vi "OPC UA SV Server.vi"() -> ()   [LabVIEW 2015]
uses:
  Controls/Folders to Add.ctl
  <vilib>/OPCUA/NI OPC UA Server.lvlib
  Sync Tag Class/Synchronised Tag.lvclass
  OPC UA Client Class/OPC UA Client.lvclass
  <vilib>/NI_Real-Time Target Support.lvlib
panel:
  out "Exit Error":errorcluster
  in  "Blacklist":string[](array[string])=["ForceValue", "RefersTo"]
  in  "Variable Containers":refnum<k21>[](array[refnum])=["ni.var.psp://localhost/SS_Real_Time_Variable_Library"]
  out "No of Tags":i32
  out "Folders":T1[](array[typedef])
  out "server endpoint URL":string
  out "URLs":string[](array[string])
  in  "update rate (ms)":u32=500
  in  "port":i32=4840
  out "Client error":errorcluster
  in  "stop":bool
  # "Errors\nShould be consolidated and logged/handled"
  # "Diagnostics"
  # "Control"
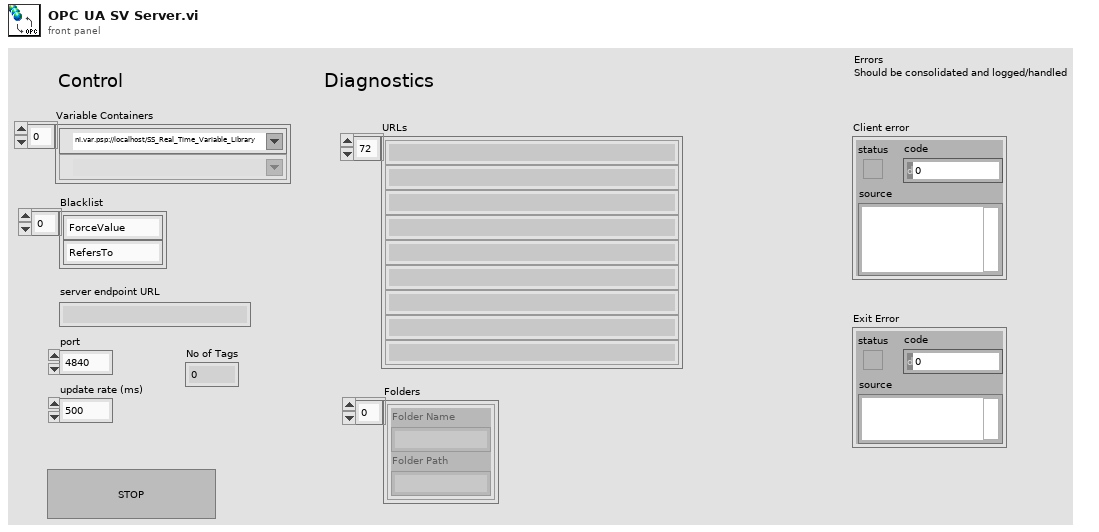
[diagram p1: front panel]
types:
  T1 = typedef "Folders to Add.ctl" = cluster{"Folder Name":string, "Folder Path":string}
  T2 = cluster{"Item URL":string, "Item Value":variant, "Timestamp":timestamp, "DataType":u32, "status code":u32}[]
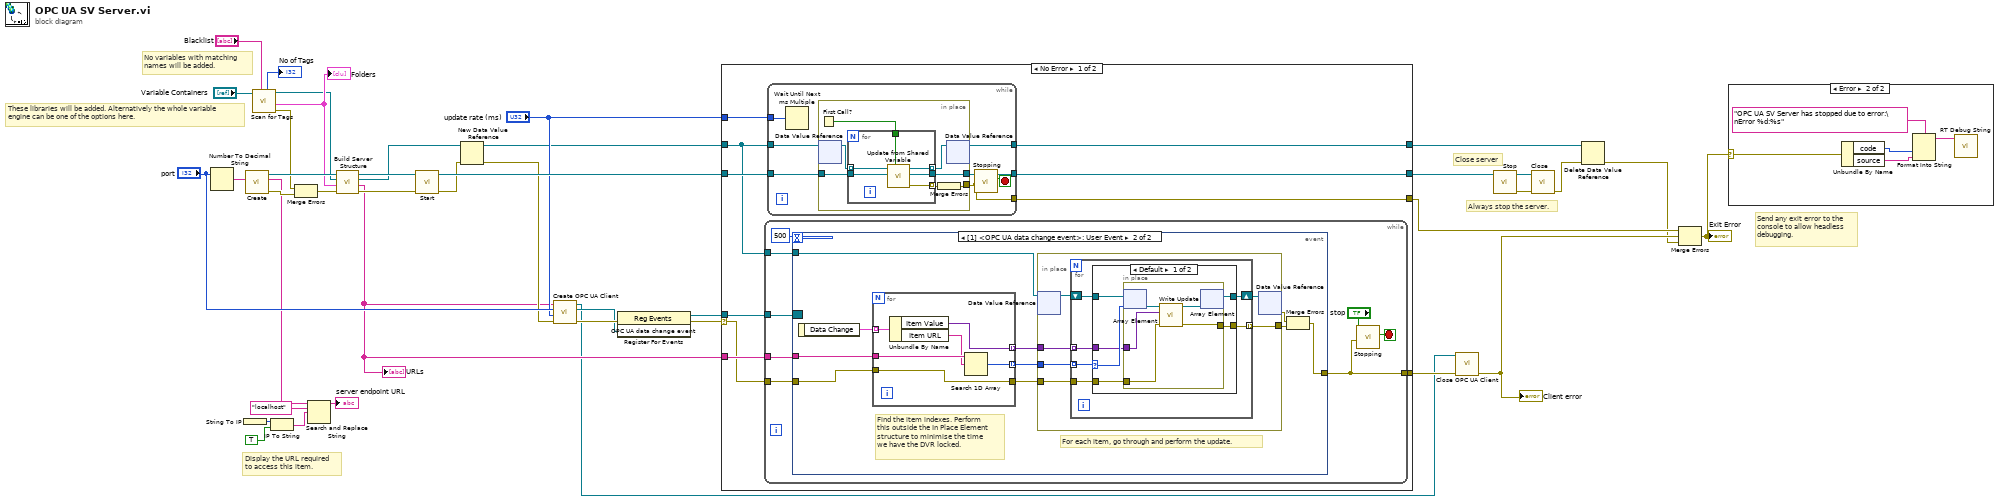
[diagram p0: block diagram]
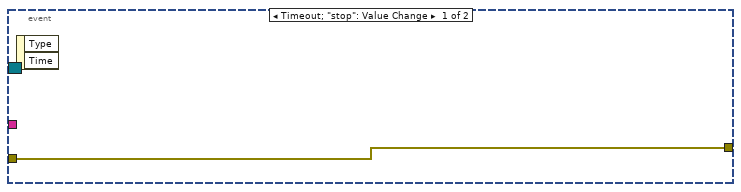
[diagram p3: hidden frame]
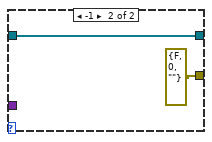
[diagram p4: hidden frame]
diagram:
  # "Send any exit error to the\nconsole to allow headless\ndebugging."
  # "Always stop the server."
  # "Display the URL required\nto access this item."
  # "Close server"
  # "These libraries will be added. Alternatively the whole variable\nengine can be one of the options here."
  # "No variables with matching\nnames will be added."
  n1 = Number To Decimal String(number="port") -> (decimal integer string=w40:string)  [unwired: 1 in]
  n2 = String To IP() -> (0:w24:u32)  [unwired: 1 in]
  n3 = call <vilib>:"Create.vi"("TCP port (49580)"=w40) -> ("error out"=w36:errorcluster, "server endpoint URL"=w29:string, "OPC UA server refnum out"=w37:refnum<k21>)  [unwired: 8 in]
  n4 = call "Scan for Tags.vi"("Blacklist"="Blacklist", "Variable Containers"="Variable Containers") -> ("error out"=w8:errorcluster, "Top Level Folders Out"=w35:T1[], "Sync Tag Array"=w23:refnum<class "Synchronised Tag.lvclass">[], "Number of Tags"=→"No of Tags":i32)  [unwired: 6 in]
  "Folders" <- w35
  n5 = IP To String(1:TRUE ("dot notation? (F)"), 2:w24) -> (0:w26:string)
  n6 = Merge Errors(w8, w36) -> (w9:errorcluster)
  n7 = Search and Replace String(input string=w29, search string="localhost", replace string=w26) -> (result string=→"server endpoint URL":string)  [unwired: 5 in, 3 out]
  n8 = call "Build Server Structure.vi"("error in (no error)"=w9, "Folders"=w35, "Tag Array In"=w23, "OPC UA server refnum in"=w37) -> ("error out"=w13:errorcluster, "URLs"=w6:string[], "Tag Array Out"=w21:refnum<class "Synchronised Tag.lvclass">[], "OPC UA server refnum out"=w34:refnum<k21>)  [unwired: 4 in]
  "URLs" <- w6
  n9 = call <vilib>:"Start.vi"("error in (no error)"=w13, "OPC UA server refnum in"=w34) -> ("error out"=w12:errorcluster, "OPC UA server refnum out"=w33:refnum<k21>)  [unwired: 8 in]
  n10 = New Data Value Reference(data value=w21, error in=w12) -> (data value reference=w20:refnum<data-value>, error out=w11:errorcluster)
  n11 = call "Create OPC UA Client.vi"("error in (no error)"=w11, "update rate (1000 ms)"="update rate (ms)", "port (4840)"="port", "URLs"=w6) -> ("error out"=w15:errorcluster, "OPC UA data change event"=w7:refnum<user-event>, "OPC UA Client.lvclass"=w5:refnum<class "OPC UA Client.lvclass">)  [unwired: 5 in]
  n12 = register-events(error in=w15, w7) -> (reference out=w41:refnum<event-registration>, error out=w14:errorcluster)  [unwired: 1 in]
  n13 = case shown="No Error" w14 {
    selector: w14 -> [w43 w122]
    tunnel: w41 -> [w51 _]
    tunnel: w33 -> [w50 w123]
    tunnel: "update rate (ms)" -> [w49 _]
    tunnel: [w48 w122] -> w30
    tunnel: w6 -> [w47 _]
    tunnel: [w46 w123] -> w22
    tunnel: w20 -> [w45 w124]
    tunnel: [w44 w124] -> w16
    tunnel: [w42 w122] -> w4
    frame No Error {
      n14 = while {
        tunnel: w51 -> [w79]
        tunnel: w47 -> [w77]
        tunnel: w43 -> [w76]
        tunnel: [w75] -> w48
        tunnel: w45 -> [w72]
        stop <- w74 stop-if-true
        n15 = event shown="[1] <OPC UA data change event>: User Event" {
          selector: w79 -> [_ _]
          dyn-events: _ -> [_ _]
          timeout: 500 -> [_ _]
          tunnel: w77 -> [_ w89]
          tunnel: w76 -> [w80 w88]
          tunnel: [w80 w81] -> w75
          tunnel: w72 -> [_ w87]
          event Timeout; "stop": Value Change {
            n16 = event-data() -> ()  [unwired: 1 in, 2 out]
          }
          event User Event {
            # "For each item, go through and perform the update."
            # "Find the item indexes. Perform\nthis outside the In Place Element\nstructure to minimise the time\nwe have the DVR locked."
            n17 = event-data() -> ("Data Change"=w90:T2)  [unwired: 1 in]
            n18 = for {
              tunnel: w90 -> [w121] mode=indexing
              tunnel: w89 -> [w120]
              tunnel: [w116] -> w84
              tunnel: w88 -> [w116]
              tunnel: [w118] -> w86 mode=indexing
              tunnel: [w117] -> w85 mode=indexing
              n19 = Unbundle By Name(w121) -> ("Item Value"=w118:variant, "Item URL"=w119:string)
              n20 = Search 1D Array(1D array=w120, element=w119) -> (index of element=w117:i32)  [unwired: 1 in]
            }
            n21 = in-place {
              in-place-border: w86 -> [w93]
              in-place-border: w85 -> [w94]
              in-place-border: w84 -> [w92]
              in-place-border: [w91] -> w82
              n22 = in-place-dvr #1(w87) -> (w96:refnum<class "Synchronised Tag.lvclass">[])  [unwired: 1 out]
              n23 = for {
                shift-right: [w101] -> w95
                shift-left: w96 -> [w100]
                tunnel: w94 -> [w102] mode=indexing
                tunnel: w93 -> [w99] mode=indexing
                tunnel: w92 -> [w98]
                tunnel: [w97] -> w91 mode=indexing
                n24 = case shown="Default" w102 {
                  selector: w102 -> [w107 _]
                  tunnel: [w106 w115] -> w101
                  tunnel: w100 -> [w108 w115]
                  tunnel: w99 -> [w105 _]
                  tunnel: w98 -> [w104 _]
                  tunnel: [w103 errorcluster {"status"=FALSE, "code"=0, "source"=""} ("error out")] -> w97
                  frame Default {
                    n25 = in-place {
                      in-place-border: w105 -> [w111]
                      in-place-border: w104 -> [w110]
                      in-place-border: [w109] -> w103
                      n26 = in-place-array #2(w108, w107) -> (w113:refnum<class "Synchronised Tag.lvclass">)
                      n27 = call "Write Update.vi"("error in (no error)"=w110, "New Value"=w111, "Sync Tag In"=w113) -> ("error out"=w109:errorcluster, "Sync Tag Out"=w112:refnum<class "Synchronised Tag.lvclass">)  [unwired: 7 in]
                      n28 = in-place-array #2(w112) -> (w106:refnum<class "Synchronised Tag.lvclass">[])  [unwired: 1 out]
                    }
                  }
                  frame -1 {
                  }
                }
              }
              n29 = in-place-dvr #1(w95) -> (w83:errorcluster)  [unwired: 1 out]
            }
            n30 = Merge Errors(w83, w82) -> (w81:errorcluster)
          }
        }
        n31 = call "Stopping.vi"("error in"=w75, "Stop"="stop") -> ("Stopping"=w74:bool)  [unwired: 8 in, 1 out]
      }
      n32 = while {
        tunnel: w49 -> [w58]
        tunnel: w45 -> [w54]
        tunnel: w50 -> [w56]
        tunnel: [w55] -> w46
        tunnel: [w53] -> w44
        tunnel: [w52] -> w42
        stop <- w57 stop-if-true
        n33 = Wait Until Next ms Multiple(millisecond multiple=w58) -> ()  [unwired: 1 out]
        n34 = in-place {
          in-place-border: w56 -> [w64]
          in-place-border: [w62] -> w52
          in-place-border: [w61] -> w55
          n35 = First Call?() -> (First Call?: T/F=w63:bool)
          n36 = in-place-dvr #3(w54) -> (w60:refnum<class "Synchronised Tag.lvclass">[])  [unwired: 1 out]
          n37 = for {
            tunnel: [w69] -> w65 mode=indexing
            tunnel: w60 -> [w71] mode=indexing
            tunnel: w64 -> [w70]
            tunnel: w63 -> [w68]
            tunnel: [w67] -> w61
            tunnel: [w66] -> w59 mode=indexing
            n38 = call "Update from Shared Variable.vi"("Force Write (F)"=w68, "OPC UA server refnum in"=w70, "SV Sync Tag"=w71) -> ("error out"=w69:errorcluster, "OPC UA server refnum out"=w67:refnum<k21>, "SV Sync Tag Out"=w66:refnum<class "Synchronised Tag.lvclass">)  [unwired: 6 in]
          }
          n39 = Merge Errors(w65) -> (w62:errorcluster)
          n40 = in-place-dvr #3(w59) -> (w53:refnum<data-value>)  [unwired: 1 out]
        }
        n41 = call "Stopping.vi"("error in"=w52) -> ("Stopping"=w57:bool)  [unwired: 9 in, 1 out]
      }
    }
    frame Error {
      # "Any error in initialisation then do not start the server."
    }
  }
  n42 = call "Close OPC UA Client.vi"("error in (no error)"=w30, "OPC UA Client.lvclass"=w5) -> ("error out"=w3:errorcluster)  [unwired: 9 in]
  "Client error" <- w3
  n43 = call <vilib>:"Stop.vi"("OPC UA server refnum in"=w22) -> ("error out"=w18:errorcluster, "OPC UA server refnum out"=w19:refnum<k21>)  [unwired: 9 in]
  n44 = call <vilib>:"Close.vi"("error in (no error)"=w18, "OPC UA server refnum in"=w19) -> ("error out"=w17:errorcluster)  [unwired: 9 in]
  n45 = Delete Data Value Reference(data value reference=w16, error in=w17) -> (error out=w2:errorcluster)  [unwired: 1 out]
  n46 = Merge Errors(w4, w3, w2) -> (w1:errorcluster)
  "Exit Error" <- w1
  n47 = case shown="Error" w1 {
    selector: w1 -> [_ w127]
    frame No Error {
    }
    frame Error {
      n48 = Unbundle By Name(w127) -> ("code"=w126:i32, "source"=w125:string)
      n49 = Format Into String(format string="OPC UA SV Server has stopped due to error:\nError %d:%s", w126, w125) -> (resulting string=w129:string)  [unwired: 2 in, 1 out]
      n50 = call <vilib>:"RT Debug String.vi"("String to write"=w129) -> ()  [unwired: 10 in, 1 out]
    }
  }
